vi "MainConfiguration.vi"(0 "NI-845X Config":cluster{"i2c configuration":T1, "Refnum in":T2}={"i2c configuration"=refnum, "Refnum in"="USB0::0x3923::0x7514::019441AA::RAW"}, 1 "AD5933 Configuration":T4={"Start Frequency / Hz"=1000.0, "Frequency Increment / Hz"=1000.0, "Number of Increments / #"=100, "Number of Setting Time Cycles / # "=200, "Exitation Voltage"=enum."2V", "PGA Gain"=enum."1x"} {"Number of Setting Time Cycles / #" max=2044 step=1; "Number of Increments / #" max=511; "Frequency Increment / Hz" min=0.1 max=100000.0 step=0.1 format="%#_6p"; "Start Frequency / Hz" min=0.0 max=100000.0 step=0.1 format="%#_6p"}, 2 "Measurement \nConfiguration":T3={"File Path"=path "", "Sampling Rate [s]"=1.0, "SaveMeas"=FALSE, "Frequencies"=[], "refnum out"=refnum} {"Sampling Rate [s]" min=1.0}, 3 "error in (no error)":errorcluster) -> (4 "AD5933 Configuration Out":T4={"Start Frequency / Hz"=1000.0, "Frequency Increment / Hz"=1000.0, "Number of Increments / #"=100, "Number of Setting Time Cycles / # "=200, "Exitation Voltage"=enum."2V", "PGA Gain"=enum."1x"} {"Number of Setting Time Cycles / #" max=2044 step=1; "Number of Increments / #" max=511; "Frequency Increment / Hz" min=0.1 max=100000.0 step=0.1 format="%#_6p"; "Start Frequency / Hz" min=0.0 max=100000.0 step=0.1 format="%#_6p"}, 5 "NI-845X Config Out":cluster{"i2c configuration":T1, "Refnum in":T2}={"i2c configuration"=refnum, "Refnum in"="USB0::0x3923::0x7514::019441AA::RAW"}, 6 "New Setup":bool, 7 "Measurement \nConfiguration out":T3={"File Path"=path "", "Sampling Rate [s]"=1.0, "SaveMeas"=FALSE, "Frequencies"=[], "refnum out"=refnum} {"Sampling Rate [s]" min=1.0}, 8 "error out":errorcluster)   [LabVIEW 2017]
uses:
  <vilib>/ni845x/ni845x.llb/ni845xControl.ctl
  TypeDefs/AD5933_Config.ctl
  <vilib>/ni845x/ni845x.llb/ni845xI2cConfiguration.ctl
  TypeDefs/MeasurementConfig.ctl
  <resource>/objmgr/NI845x.rc
panel:
  in  "Device":T2
  in  "Clock Rate (kHz)":u16=100
  in  "Use Internal I2C Pullup Resistor":bool=TRUE
  in  "I/O Voltage Level":i32(ring)=33 items=["3.3V"=33, "2.5V"=25, "1.8V"=18, "1.5V"=15, "1.2V"=12]
  in  "Set":bool
  in  "Cancel":bool
  # "NI-845X Config"
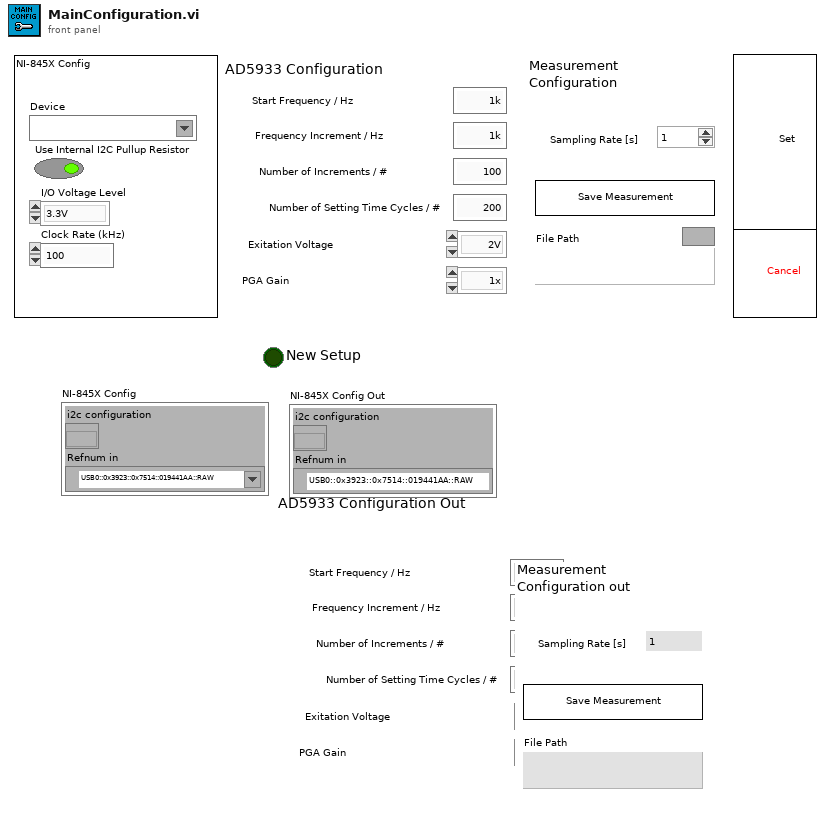
[diagram p1: front panel]
types:
  T1 = typedef "ni845xI2cConfiguration.ctl" = refnum<k20>
  T2 = typedef "ni845xControl.ctl" = refnum<k21>
  T3 = typedef "MeasurementConfig.ctl" = cluster{"File Path":path, "Sampling Rate [s]":dbl, "SaveMeas":bool, "Frequencies":dbl[], "refnum out":refnum<file>}
  T4 = typedef "AD5933_Config.ctl" = cluster{"Start Frequency / Hz":dbl, "Frequency Increment / Hz":dbl, "Number of Increments / #":u16, "Number of Setting Time Cycles / # ":u16, "Exitation Voltage":enum8{"2V", "200mV", "400mV", "1V"}, "PGA Gain":enum8{"5x", "1x"}}
  T5 = enum16{"open", "replace", "create", "open or create", "replace or create", "replace or create with confirmation"}
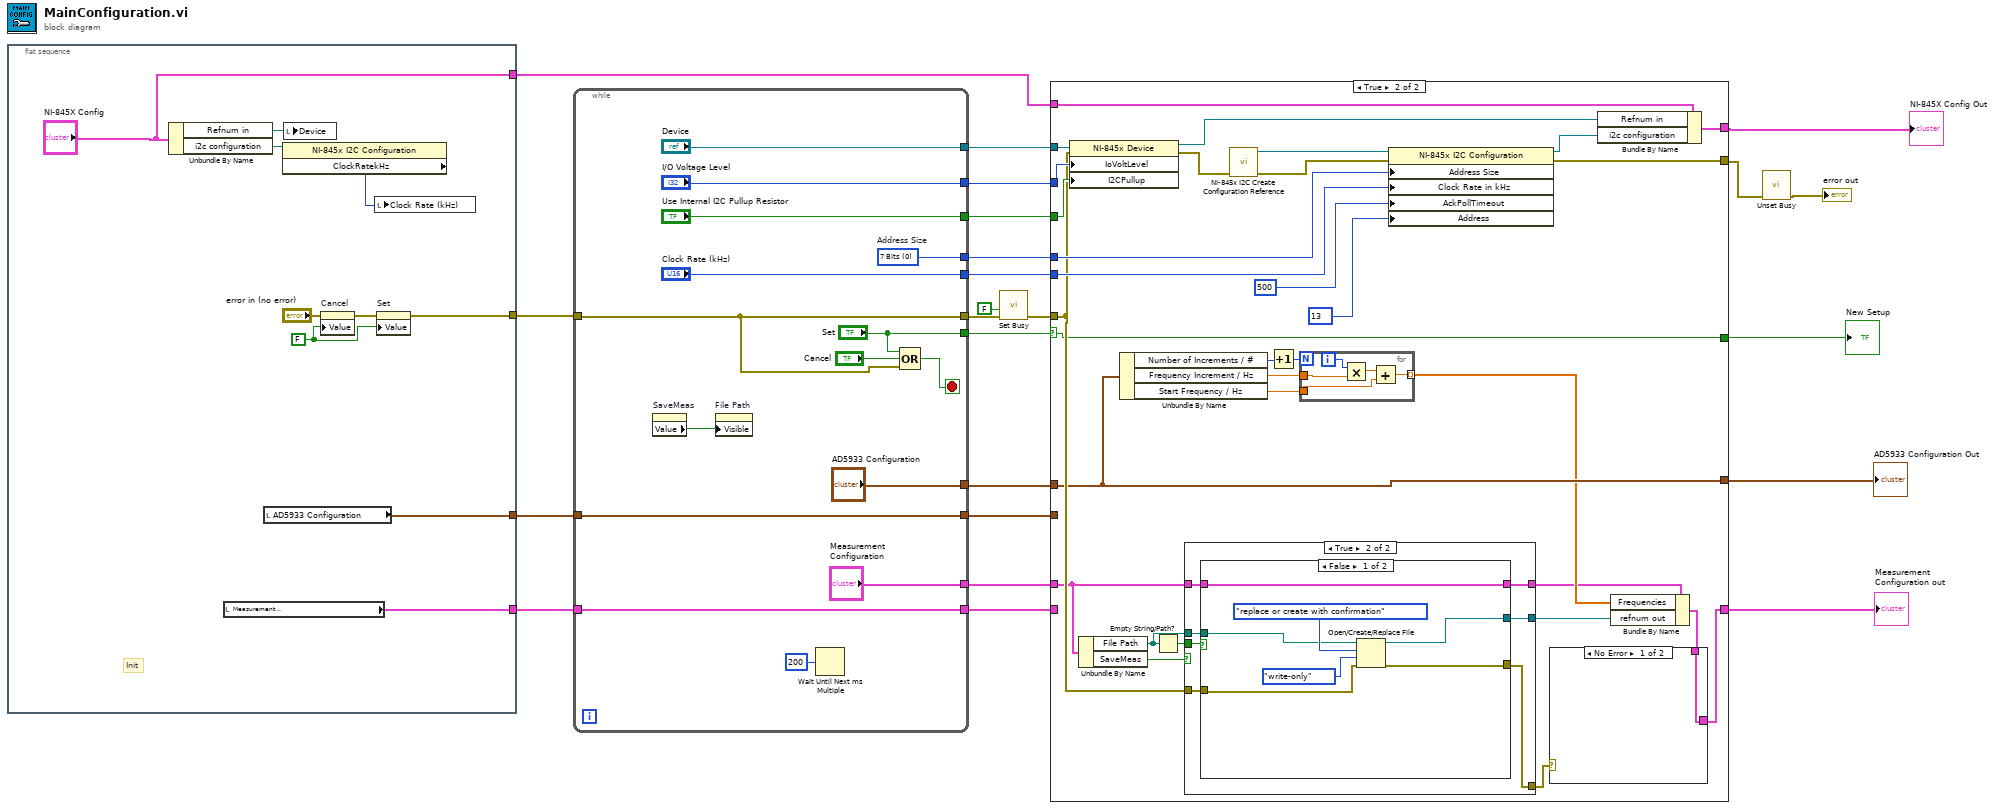
[diagram p0: block diagram]
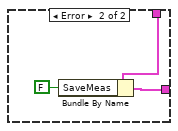
[diagram p3: hidden frame]
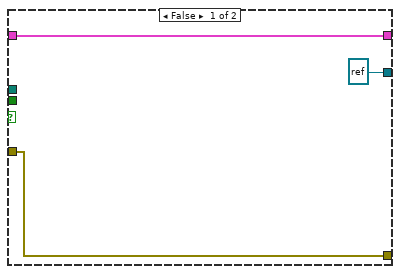
[diagram p4: hidden frame]
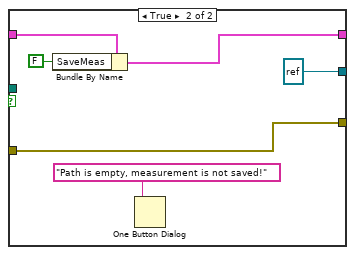
[diagram p5: hidden frame]
diagram:
  n1 = flat-sequence {
    tunnel: [w30] -> w12
    tunnel: [w29] -> w7
    tunnel: [w28] -> w6
    tunnel: ["NI-845X Config"] -> w2
    frame #0 {
      w32 = FALSE ("Cancel")
      # "Init"
      n2 = Unbundle By Name("NI-845X Config") -> ("Refnum in"=w25:T2, "i2c configuration"=w27:T1)
      n3 = local read "Measurement \nConfiguration"() -> (w28:T3)
      n4 = local read "AD5933 Configuration"() -> (w29:T4)
      n5 = property class="NI-845x I2C Configuration"(reference=w27) -> ("ClockRatekHz"=w26:u16)  [unwired: 1 in, 2 out]
      n6 = local write "Device"(w25) -> ()
      n7 = property on="Cancel" class="Bool (strict)"(error in="error in (no error)", "Value"=w32) -> (error out=w33:errorcluster)  [unwired: 1 in, 1 out]
      n8 = local write "Clock Rate (kHz)"(w26) -> ()
      n9 = property on="Set" class="Bool (strict)"(error in=w33, "Value"=w32) -> (error out=w30:errorcluster)  [unwired: 1 in, 1 out]
    }
  }
  n10 = while {
    tunnel: ["Clock Rate (kHz)"] -> w23
    tunnel: [w47] -> w22
    tunnel: ["Device"] -> w21
    tunnel: ["I/O Voltage Level"] -> w20
    tunnel: ["Use Internal I2C Pullup Resistor"] -> w19
    tunnel: ["Set"] -> w18
    tunnel: [w40] -> w16
    tunnel: w12 -> [w40]
    tunnel: ["AD5933 Configuration"] -> w9
    tunnel: [w39] -> w8
    tunnel: w7 -> [w39]
    tunnel: w6 -> [w34]
    tunnel: ["Measurement \nConfiguration"] -> w5
    tunnel: [w34] -> w3
    stop <- w43 stop-if-true
    w47 = 0 items=["7 Bits", "10 Bits"]  # Address Size
    n11 = property on="SaveMeas" class="Bool (strict)"() -> ("Value"=w37:bool)  [unwired: 2 in, 2 out]
    n12 = property on="File Path" class="Path"("Visible"=w37) -> ()  [unwired: 2 in, 2 out]
    n13 = Wait Until Next ms Multiple(millisecond multiple=u32 200) -> ()  [unwired: 1 out]
    n14 = Compound Arithmetic op=OR("Set", "Cancel", w40) -> (w43:bool)
  }
  n15 = call <vilib>:"Set Busy.vi"("error in (no error)"=w16, "disable click? (T)"=FALSE) -> ("error out"=w17:errorcluster)  [unwired: 8 in, 1 out]
  n16 = case shown="True" w18 {
    selector: w18 -> [w49 w58]
    tunnel: w23 -> [_ w85]
    tunnel: w22 -> [_ w84]
    tunnel: w21 -> [_ w81]
    tunnel: w20 -> [_ w80]
    tunnel: w19 -> [_ w79]
    tunnel: w17 -> [w53 w68]
    tunnel: [w53 w77] -> w14
    tunnel: [w51 w72] -> w11
    tunnel: w2 -> [w51 w71]
    tunnel: [w52 w63] -> w10
    tunnel: w9 -> [_ w63]
    tunnel: w8 -> [w52 _]
    tunnel: [w50 w54] -> w4
    tunnel: w5 -> [_ w61]
    tunnel: w3 -> [w50 _]
    tunnel: [w49 w58] -> w1
    frame False {
    }
    frame True {
      n17 = property on="Property Node" class="NI-845x Device"(reference=w81, error in=w68, "IoVoltLevel"=w80, "I2CPullup"=w79) -> (reference out=w73:T2, error out=w78:errorcluster)
      n18 = Unbundle By Name(w61) -> ("File Path"=w62:path, "SaveMeas"=w70:bool)
      n19 = Unbundle By Name(w63) -> ("Number of Increments / #"=w66:u16, "Frequency Increment / Hz"=w64:dbl, "Start Frequency / Hz"=w65:dbl)
      n20 = Empty String/Path?(string/path=w62) -> (empty?=w69:bool)
      n21 = case shown="True" w70 {
        tunnel: w69 -> [_ w104]
        tunnel: w68 -> [w97 w103]
        tunnel: w62 -> [_ w102]
        tunnel: [w97 w101] -> w57
        tunnel: w61 -> [w96 w100]
        tunnel: [w96 w99] -> w56
        tunnel: [refnum<file> refnum ("refnum out") w98] -> w60
        frame False {
        }
        frame True {
          n22 = case shown="False" w104 {
            tunnel: w103 -> [w109 w115]
            tunnel: w102 -> [w108 _]
            tunnel: [w107 refnum<file> refnum ("refnum out")] -> w98
            tunnel: [w106 w115] -> w101
            tunnel: w100 -> [w105 w114]
            tunnel: [w105 w113] -> w99
            frame False {
              n23 = Open/Create/Replace File(file path (use dialog)=w108, error in=w109, operation (0:open)=T5."replace or create with confirmation", access (0:read/write)=enum16{"read/write", "read-only", "write-only"}."write-only") -> (refnum out=w107:refnum<file>, error out=w106:errorcluster)  [unwired: 2 in, 1 out]
            }
            frame True {
              n24 = Bundle By Name(cluster=w114, "SaveMeas"=FALSE) -> (w113:T3)
              n25 = One Button Dialog(message="Path is empty, measurement is not saved!") -> ()  [unwired: 1 in, 1 out]
            }
          }
        }
      }
      n26 = call <vilib>:"NI-845x I2C Create Configuration Reference.vi"("error in (no error)"=w78) -> ("error out"=w82:errorcluster, "i2c configuration"=w83:T1)  [unwired: 9 out]
      n27 = Increment(x=w66) -> (x+1=w67:u16)
      n28 = for {
        N: w67 -> [_]
        tunnel: w64 -> [w93]
        tunnel: w65 -> [w92]
        tunnel: [w91] -> w59 mode=indexing
        i -> [w90]
        n29 = Multiply(x=w90, y=w93) -> (x*y=w94:dbl)
        n30 = Add(x=w94, y=w92) -> (x+y=w91:dbl)
      }
      n31 = property class="NI-845x I2C Configuration"(reference=w83, error in=w82, "Address Size"=w84, "Clock Rate in kHz"=w85, "AckPollTimeout"=u16 500 ("ACK Poll Timeout"), "Address"=u16 13) -> (reference out=w74:T1, error out=w77:errorcluster)
      n32 = Bundle By Name(cluster=w71, "Refnum in"=w73, "i2c configuration"=w74) -> (w72:cluster{"i2c configuration":T1, "Refnum in":T2})
      n33 = Bundle By Name(cluster=w56, "Frequencies"=w59, "refnum out"=w60) -> (w55:T3)
      n34 = case shown="No Error" w57 {
        tunnel: w55 -> [w86 w88]
        tunnel: [w86 w87] -> w54
        frame No Error {
        }
        frame Error {
          n35 = Bundle By Name(cluster=w88, "SaveMeas"=FALSE) -> (w87:T3)
        }
      }
    }
  }
  "AD5933 Configuration Out" <- w10
  "NI-845X Config Out" <- w11
  "Measurement \nConfiguration out" <- w4
  "New Setup" <- w1
  n36 = call <vilib>:"Unset Busy.vi"("error in (no error)"=w14) -> ("error out"=→"error out":errorcluster)  [unwired: 10 in]
